vi "p284.vi"() -> ()   [LabVIEW 2017]
panel:
  out "Boolean":bool
  in  "stop 2":bool
  in  "stop":bool
  in  "String 2":string
  out "String":string
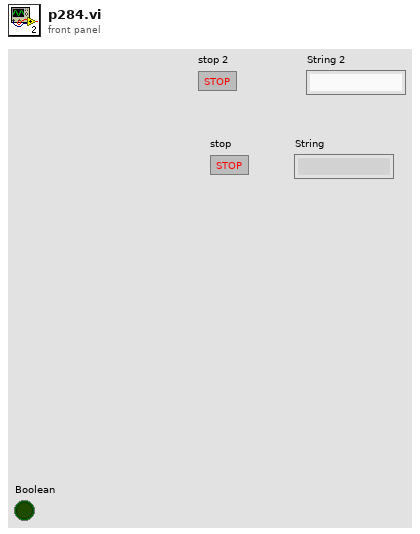
[diagram p1: front panel]
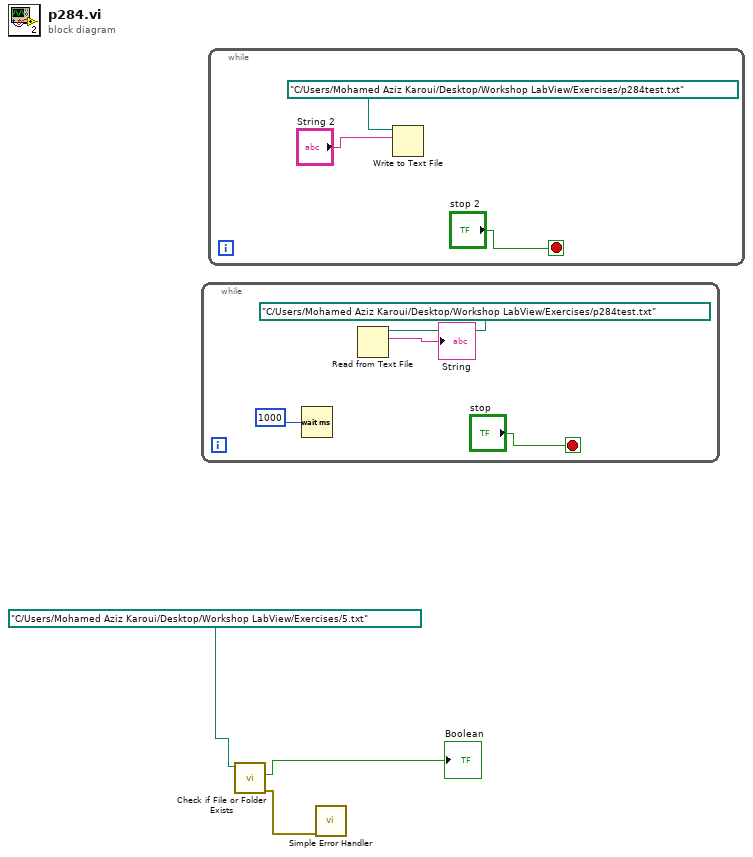
[diagram p0: block diagram]
diagram:
  n1 = while {
    stop <- "stop" stop-if-true
    n2 = Wait (ms)(milliseconds to wait=1000) -> ()  [unwired: 1 out]
    n3 = Read from Text File(file (use dialog)=path "C:/Users/Mohamed Aziz Karoui/Desktop/Workshop LabView/Exercises/p284test.txt") -> (text=→"String":string)  [unwired: 3 in, 3 out]
  }
  n4 = while {
    stop <- "stop 2" stop-if-true
    n5 = Write to Text File(file (use dialog)=path "C:/Users/Mohamed Aziz Karoui/Desktop/Workshop LabView/Exercises/p284test.txt", text="String 2") -> ()  [unwired: 2 in, 3 out]
  }
  n6 = call <vilib>:"Check if File or Folder Exists.vi"("path"=path "C:/Users/Mohamed Aziz Karoui/Desktop/Workshop LabView/Exercises/5.txt") -> ("error out"=w3:errorcluster, "file or folder exists?"=→"Boolean":bool)  [unwired: 8 in, 1 out]
  n7 = call <vilib>:"Simple Error Handler.vi"("error in (no error)"=w3) -> ()  [unwired: 4 in, 5 out]
